vi "main.vi"() -> ()   [LabVIEW 2023]
panel:
  in  "Bereichsumschaltung":dbl(knob) scale=0.1..5.0
  out "?":dbl(slide) scale=0.1..5.0 scale format="%#.1g"
  in  "?":bool
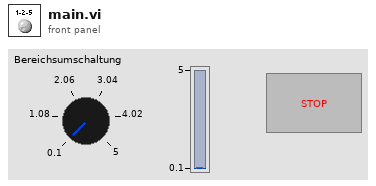
[diagram p1: front panel]
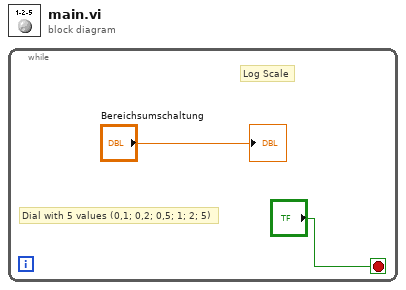
[diagram p0: block diagram]
diagram:
  n1 = while {
    stop <- "?" stop-if-true
    # "Log Scale"
    # "Dial with 5 values (0,1; 0,2; 0,5; 1; 2; 5)"
    "?" <- "Bereichsumschaltung"
  }
